vi "Check for errors.vi"(8 "error in":errorcluster, 11 "Next state in":T1) -> (0 "error out":errorcluster, 3 "Next state out":T1)   [LabVIEW 2023]
uses:
  States.ctl
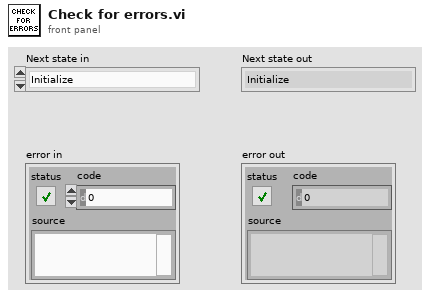
[diagram p1: front panel]
types:
  T1 = typedef "States.ctl" = enum16{"Initialize", "Select Variant", "Idle", "Start Test", "Test", "Result", "Deinitialize"}
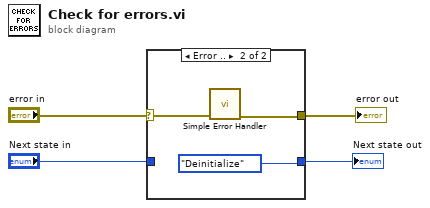
[diagram p0: block diagram]
diagram:
  n1 = case shown="Error .." "error in" {
    selector: "error in" -> [w5 w8]
    tunnel: "Next state in" -> [w6 _]
    tunnel: [w6 States."Deinitialize"] -> w2
    tunnel: [w5 w7] -> w1
    frame No Error {
    }
    frame Error {
      n2 = call <vilib>:"Simple Error Handler.vi"("error in (no error)"=w8) -> ("error out"=w7:errorcluster)  [unwired: 4 in, 4 out]
    }
  }
  "Next state out" <- w2
  "error out" <- w1
